vi "GVmotor_convert_voltage_to_turn.vi"(6 "v0":dbl format="%#_13g", 7 "coef":dbl=0.309 format="%#_13g", 8 "status_in":bool=TRUE, 11 "voltage":dbl) -> (0 "status_out":bool=TRUE, 2 "percent":dbl caption="%", 3 "turn":dbl)   [LabVIEW 2019]
panel:
  # "1/4 valve turns = 1/2 pot turns.\n3 pot turns = 5 V.\nThus 1 V = 0.3 valve turn."
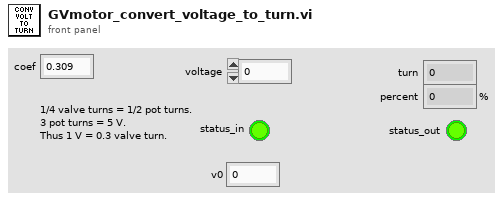
[diagram p1: front panel]
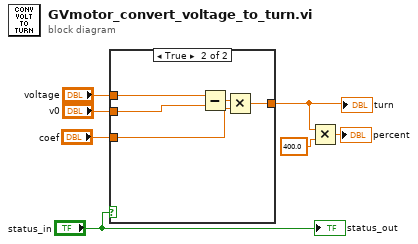
[diagram p0: block diagram]
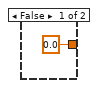
[diagram p2: hidden frame]
diagram:
  n1 = case shown="True" "status_in" {
    tunnel: [0.0 w12] -> w2
    tunnel: "voltage" -> [_ w11]
    tunnel: "v0" -> [_ w10]
    tunnel: "coef" -> [_ w9]
    frame False {
    }
    frame True {
      n2 = Subtract(x=w11, y=w10) -> (x-y=w13:dbl)
      n3 = Multiply(x=w13, y=w9) -> (x*y=w12:dbl)
    }
  }
  "turn" <- w2
  n4 = Multiply(x=w2, y=400.0) -> (x*y=→"percent":dbl)
  "status_out" <- "status_in"
